vi "Increment counter.vi"(8 "error in (no error)":errorcluster, 11 "Counter name (dflt=blank)":string) -> (0 "error out":errorcluster, 3 "Value (after increment)":i32)   [LabVIEW 2021, in "Named Counters.lvlib"]
uses:
  Named Counters.lvlib
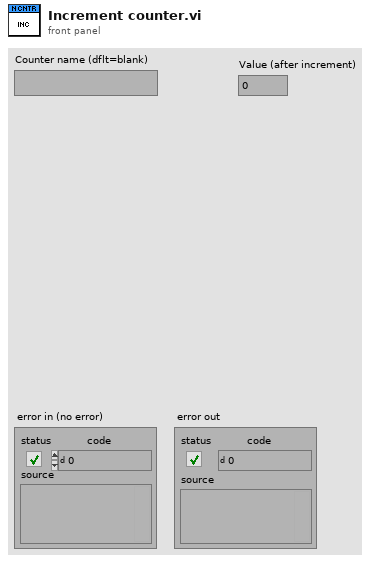
[diagram p1: front panel]
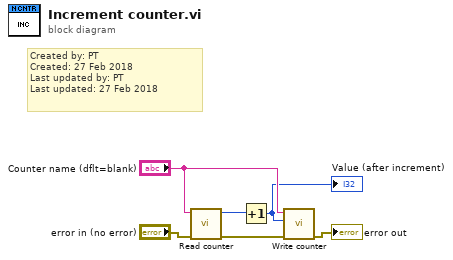
[diagram p0: block diagram]
diagram:
  # "Created by: PT\nCreated: 27 Feb 2018\nLast updated by: PT\nLast updated: 27 Feb 2018"
  n1 = call "Read counter.vi"("error in (no error)"="error in (no error)", "Counter name (dflt=blank)"="Counter name (dflt=blank)") -> ("error out"=w4:errorcluster, "Value"=w3:i32)  [unwired: 8 in]
  n2 = Increment(x=w3) -> (x+1=w1:i32)
  "Value (after increment)" <- w1
  n3 = call "Write counter.vi"("error in (no error)"=w4, "Value"=w1, "Counter name (dflt=blank)"="Counter name (dflt=blank)") -> ("error out"=→"error out":errorcluster)  [unwired: 8 in]
